vi "displayConfigurableElements.vi"(11 "ConfigurationThisComponent in":refnum<class "ConfigurationTestParameters.lvclass">) -> (3 "ConfigurationThisComponent out":refnum<class "ConfigurationTestParameters.lvclass">)   [LabVIEW 2015, in "ConfigurationTestParameters.lvclass"]
uses:
  ConfigurationTestParameters.lvclass
  <userlib>/Common/Log/Config/Log.ctl
  Typedefs/Supply Voltage Tests.ctl
  Typedefs/Supply Voltage Test.ctl
  Typedefs/ILC Analog Output Tests.ctl
  Typedefs/ILC Static Analog Output Test.ctl
  Typedefs/ILC Analog Output Test.ctl
  Typedefs/Test Values.ctl
  Typedefs/ILC EXC Analog Output Test.ctl
  Typedefs/ILC DAC Analog Output Test.ctl
  Typedefs/ILC Analog Input Tests.ctl
  Typedefs/AI Voltage to NI Voltage.ctl
  Typedefs/ILC Ch0 Analog Input Test.ctl
  Typedefs/Multichannel Analog Input Test.ctl
  Typedefs/Device Configuration Tests.ctl
  Typedefs/1-Wire Test.ctl
  Typedefs/ILC Digital Input Tests.ctl
  Typedefs/ILC Digital Input Test.ctl
  Typedefs/ILC GPI Digital Input Test.ctl
  Typedefs/ILC Digital Output Tests.ctl
  Typedefs/ILC Digital Output Test.ctl
  Typedefs/Digital Signal Level.ctl
  Typedefs/UART Serial Test.ctl
  Typedefs/MUX Settings.ctl
  Typedefs/SSI Serial Test.ctl
  Typedefs/Ground Test.ctl
  Typedefs/ILC Static Digital Output Test.ctl
  Typedefs/Motor Drive Test.ctl
  <userlib>/Common/Log/Log.lvlib
  Typedefs/ILCBTTypedefs.lvlib
panel:
  in  "ctrlRefArrayUsrEvnt":refnum<user-event>
  in  "ConfigTab":T1(tab)
  in  "TestDataLog":T2={"Log Directory"=path "", "Log Filename Base"="", "Max records per file"=1000, "Comment"=""} {"Max records per file" min=100 max=1000000}
  in  "Supply Voltage Tests":T3={"3.3 V Supply"={"Analog Supply DAQ Channel to Read"="AI3", "Digital Supply DAQ Channel to Read"="AI3", "Expected Value"=0.0, "Tolerance"=0.0}, "5 V Supply"={"Analog Supply DAQ Channel to Read"="AI3", "Digital Supply DAQ Channel to Read"="AI3", "Expected Value"=0.0, "Tolerance"=0.0}} {"5 V Supply"."Tolerance" format="%.3f"; "5 V Supply"."Expected Value" format="%.3f"; "3.3 V Supply"."Tolerance" format="%.3f"; "3.3 V Supply"."Expected Value" format="%.3f"}
  in  "Device Configuration Tests":T5
  in  "ILC Digital Input Tests":T7 {"General Purpose Digital Input"."Tachometer Values to Expect"."Stop Value" format="%.6f"; "General Purpose Digital Input"."Tachometer Values to Expect"."Start Value" format="%.6f"; "General Purpose Digital Input"."Frequency Values to Test"."Stop Value" format="%.6f"; "General Purpose Digital Input"."Frequency Values to Test"."Start Value" format="%.6f"}
  in  "ILC Digital Output Tests":T11
  in  "ILC Analog Output Tests":T20 {"DAC"."Tolerance" format="%.4f"; "DAC"."Test Values"."Stop Value" format="%.6f"; "DAC"."Test Values"."Start Value" format="%.6f"; "EXC"."Tolerance" format="%.4f"; "EXC"."Expected Value" format="%.4f"; "BIAS"."Tolerance" format="%.4f"; "BIAS"."Expected Value" format="%.4f"; "ROT"."Tolerance" format="%.4f"; "ROT"."Test Values"."Stop Value" format="%.6f"; "ROT"."Test Values"."Start Value" format="%.6f"; "Vref"."Tolerance" format="%.4f"; "Vref"."Expected Value" format="%.4f"}
  in  "ILC Analog Input Tests":T25 {"5 Channels"."Tolerance" format="%.9f"; "5 Channels"."Test Values"."Stop Value" format="%.6f"; "5 Channels"."Test Values"."Start Value" format="%.6f"; "5 Channels"."PGA Gain Coefficients" max=7; "3 Channels"."Tolerance" format="%.9f"; "3 Channels"."Test Values"."Stop Value" format="%.6f"; "3 Channels"."Test Values"."Start Value" format="%.6f"; "3 Channels"."PGA Gain Coefficients" max=7; "AO Voltage Data"."Bias" min=0.0 max=10.0 format="%.3f"; "AO Voltage Data"."NI Scaling" min=0.0 max=10.0 format="%.3f"; "AO Voltage Data"."Vref" min=0.0 max=10.0 format="%.3f"}
  # "3.3 V Supply"
  # "5 V Supply"
  # "Unique ID Test"
  # "TEDS Status Test"
  # "ms"
  # "Vref"
  # "ROT"
  # "DAC"
  # "BIAS"
  # "EXC"
  # "ms"
  # "AO Voltage Data"
  # "1 Channel"
  # "3 Channels"
  # "5 Channels"
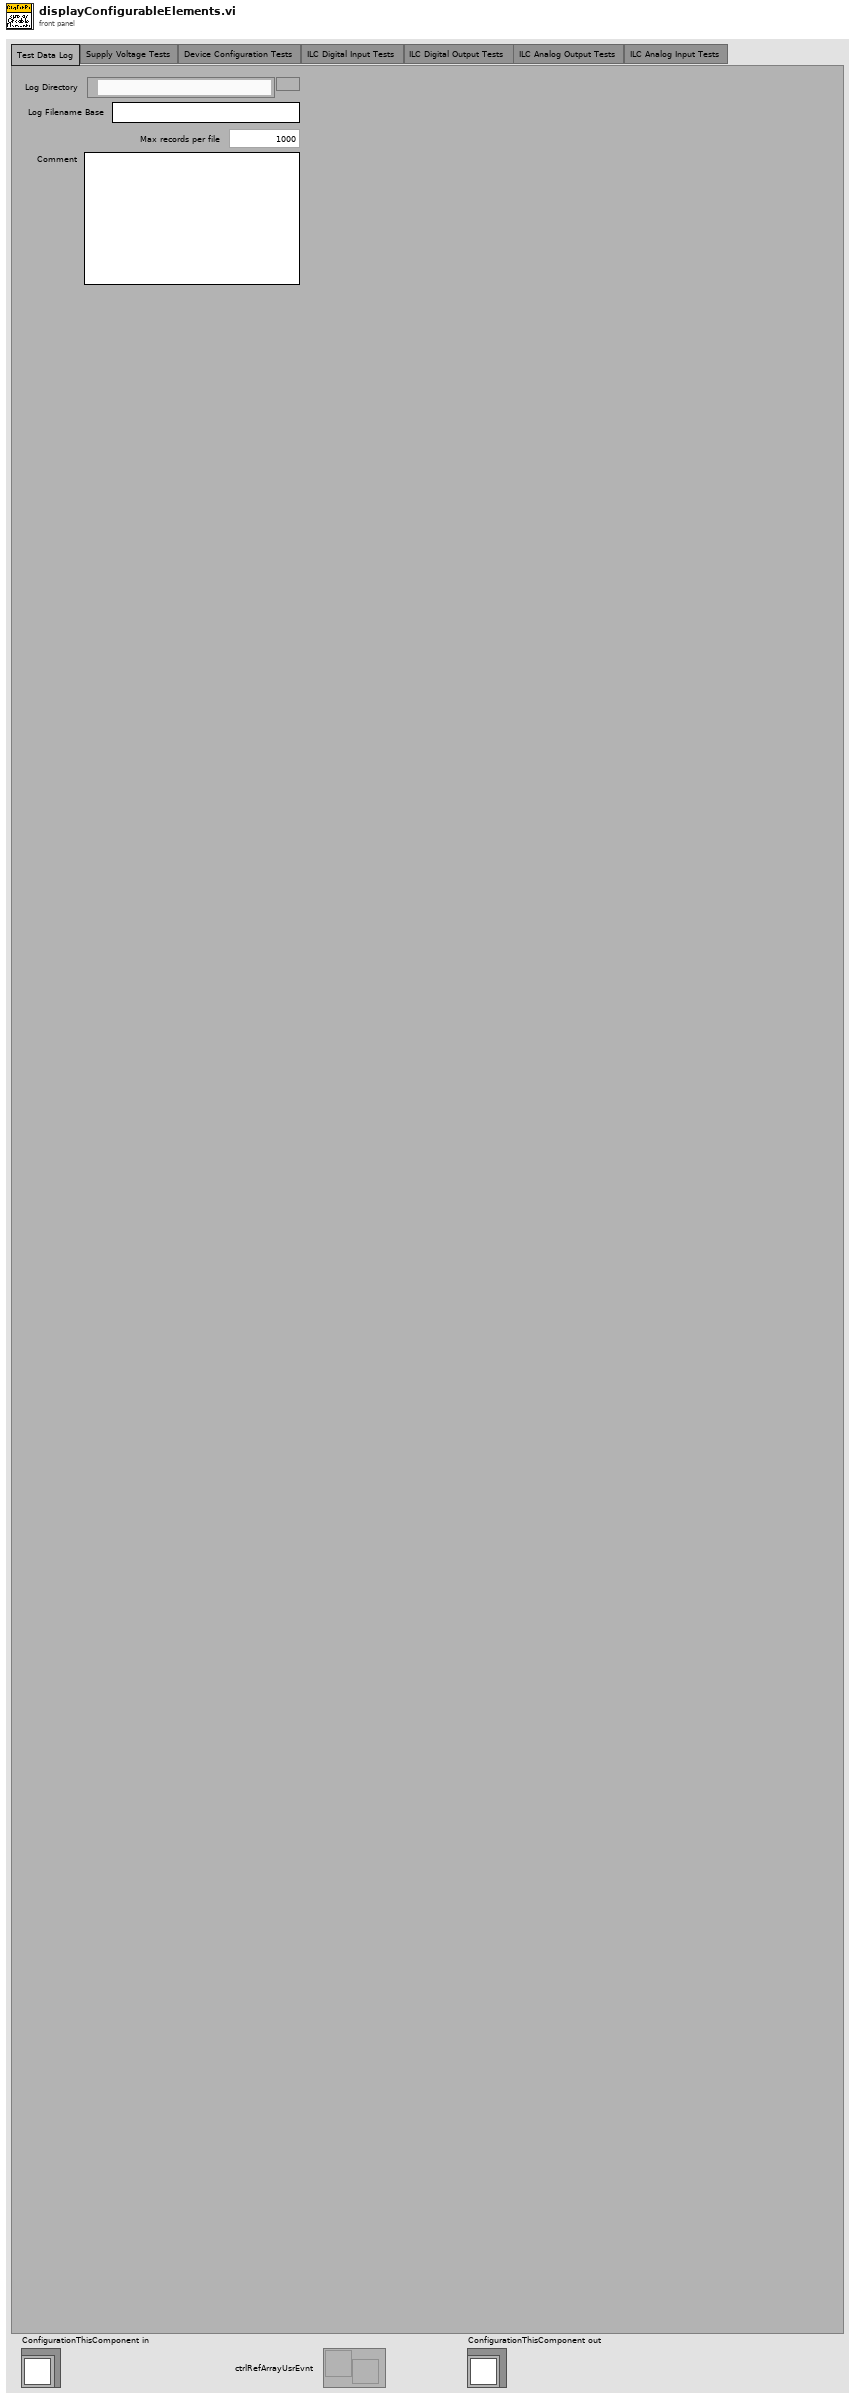
[diagram p1: front panel]
types:
  T1 = enum32{"Test Data Log", "Supply Voltage Tests", "Device Configuration Tests", "ILC Digital Input Tests", "ILC Digital Output Tests", "ILC Analog Output Tests", "ILC Analog Input Tests"}
  T2 = typedef "Log.lvlib/Log.ctl" = cluster{"Log Directory":path, "Log Filename Base":string, "Max records per file":u32, "Comment":string}
  T3 = typedef "ILCBTTypedefs.lvlib/Supply Voltage Tests.ctl" = cluster{"3.3 V Supply":T4, "5 V Supply":T4}
  T4 = typedef "ILCBTTypedefs.lvlib/Supply Voltage Test.ctl" = cluster{"Analog Supply DAQ Channel to Read":refnum<k21>, "Digital Supply DAQ Channel to Read":refnum<k21>, "Expected Value":dbl[unit], "Tolerance":dbl[unit]}
  T5 = typedef "ILCBTTypedefs.lvlib/Device Configuration Tests.ctl" = cluster{"Unique ID Test":T6, "TEDS Status Test":T6}
  T6 = typedef "ILCBTTypedefs.lvlib/1-Wire Test.ctl" = cluster{"Expected Value":string}
  T7 = typedef "ILCBTTypedefs.lvlib/ILC Digital Input Tests.ctl" = cluster{"Limit Switch 1:":T8, "Limit Switch 2:":T8, "General Purpose Digital Input":T9}
  T8 = typedef "ILCBTTypedefs.lvlib/ILC Digital Input Test.ctl" = cluster{"DAQmx Global Channel":refnum<k21>, "High Level Value to Test":enum16{"Low", "High"}, "High Level Value to Expect":enum16{"Low", "High"}, "Low Level Value to Test":enum16{"Low", "High"}, "Low Level Value to Expect":enum16{"Low", "High"}}
  T9 = typedef "ILCBTTypedefs.lvlib/ILC GPI Digital Input Test.ctl" = cluster{"DAQ Channel to Write":refnum<k21>, "Frequency Values to Test":T10, "Tachometer Values to Expect":T10}
  T10 = typedef "ILCBTTypedefs.lvlib/Test Values.ctl" = cluster{"Start Value":dbl, "Stop Value":dbl, "Number of Steps":u16}
  T11 = typedef "ILCBTTypedefs.lvlib/ILC Digital Output Tests.ctl" = cluster{"SSR":T12, "UART Serial Test":T14, "SSI Serial Test":T16, "Ground Test":T17, "Motor Drive Test":T19}
  T12 = typedef "ILCBTTypedefs.lvlib/ILC Digital Output Test.ctl" = cluster{"DAQ Channel to Read":refnum<k21>, "High Level Value to Test":T13, "High Level Value to Expect":T13, "Low Level Value to Test":T13, "Low Level Value to Expect":T13}
  T13 = typedef "ILCBTTypedefs.lvlib/Digital Signal Level.ctl" = enum16{"Low", "High"}
  T14 = typedef "ILCBTTypedefs.lvlib/UART Serial Test.ctl" = cluster{"MUX Settings":T15, "CTS":T12, "TXD":T12, "RTS":T12, "RXD":T12}
  T15 = typedef "ILCBTTypedefs.lvlib/MUX Settings.ctl" = cluster{"MUX_AO":T13, "MUX_A1":T13}
  T16 = typedef "ILCBTTypedefs.lvlib/SSI Serial Test.ctl" = cluster{"MUX Settings":T15, "Out_SS":T12, "Out_SDI":T12, "Out_SCLK":T12, "Reset":T12}
  T17 = typedef "ILCBTTypedefs.lvlib/Ground Test.ctl" = cluster{"MUX Settings":T15, "Gnd1":T18, "Gnd2":T18, "Gnd3":T18, "Gnd4":T18}
  T18 = typedef "ILCBTTypedefs.lvlib/ILC Static Digital Output Test.ctl" = cluster{"DAQ Channel to Read":refnum<k21>, "Expected Signal Level":T13}
  T19 = typedef "ILCBTTypedefs.lvlib/Motor Drive Test.ctl" = cluster{"MUX Settings":T15, "SM_CW":T12, "SM_CCW":T12, "SM_GPI":T12}
  T20 = typedef "ILCBTTypedefs.lvlib/ILC Analog Output Tests.ctl" = cluster{"Delay Between Test Steps":u16, "Vref":T21, "ROT":T22, "BIAS":T21, "EXC":T23, "DAC":T24}
  T21 = typedef "ILCBTTypedefs.lvlib/ILC Static Analog Output Test.ctl" = cluster{"DAQ Channel to Read":refnum<k21>, "Expected Value":dbl[unit], "Tolerance":dbl[unit]}
  T22 = typedef "ILCBTTypedefs.lvlib/ILC Analog Output Test.ctl" = cluster{"DAQ Channel to Read":refnum<k21>, "Test Values":T10, "Tolerance":dbl[unit]}
  T23 = typedef "ILCBTTypedefs.lvlib/ILC EXC Analog Output Test.ctl" = cluster{"EXC1 DAQ Channel to Read":refnum<k21>, "EXC2 DAQ Channel to Read":refnum<k21>, "EXC3 DAQ Channel to Read":refnum<k21>, "EXC4 DAQ Channel to Read":refnum<k21>, "Expected Value":dbl[unit], "Tolerance":dbl[unit]}
  T24 = typedef "ILCBTTypedefs.lvlib/ILC DAC Analog Output Test.ctl" = cluster{"DAC1 DAQ Channel to Read":refnum<k21>, "DAC2 DAQ Channel to Read":refnum<k21>, "DAC3 DAQ Channel to Read":refnum<k21>, "DAC4 DAQ Channel to Read":refnum<k21>, "Test Values":T10, "Tolerance":dbl[unit]}
  T25 = typedef "ILCBTTypedefs.lvlib/ILC Analog Input Tests.ctl" = cluster{"CH13 DAQ Channel to Write":refnum<k21>, "CH24 DAQ Channel to Write":refnum<k21>, "AO Voltage Data":T26, "Delay Between Test Steps":u16, "1 Channel":T27, "3 Channels":T28, "5 Channels":T28}
  T26 = typedef "ILCBTTypedefs.lvlib/AI Voltage to NI Voltage.ctl" = cluster{"ADC Bit Count":u16, "Vref":dbl[unit], "NI Scaling":dbl, "Bias":dbl[unit]}
  T27 = typedef "ILCBTTypedefs.lvlib/ILC Ch0 Analog Input Test.ctl" = cluster{"ADC Configurations":string[], "Value to Expect":i32, "Tolerance":i32}
  T28 = typedef "ILCBTTypedefs.lvlib/Multichannel Analog Input Test.ctl" = cluster{"ADC Configurations":string[], "PGA Gain Coefficients":u16[], "Test Values":T10, "Tolerance":dbl[unit]}
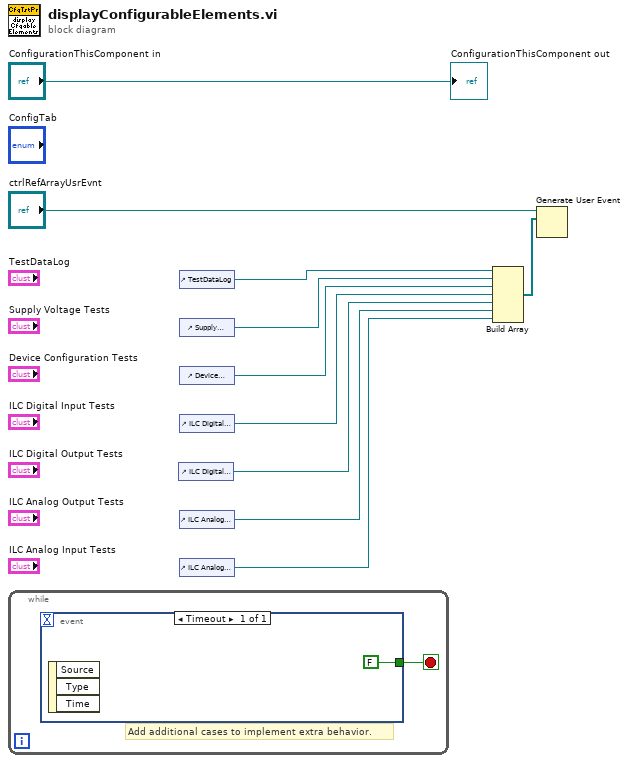
[diagram p0: block diagram]
diagram:
  n1 = while {
    stop <- w11 stop-if-true
    # "Add additional cases to implement extra behavior."
    n2 = event shown="[0] Timeout" {
      selector: _ -> [_]
      dyn-events: _ -> [_]
      timeout: _ -> [_]
      tunnel: [FALSE] -> w11
      event Timeout {
        n3 = event-data() -> ()  [unwired: 1 in, 3 out]
      }
    }
  }
  n4 = control-ref of="ILC Digital Output Tests"() -> (w3:refnum<vi>)
  n5 = control-ref of="TestDataLog"() -> (w7:refnum<vi>)
  n6 = control-ref of="Supply Voltage Tests"() -> (w6:refnum<vi>)
  n7 = control-ref of="Device Configuration Tests"() -> (w5:refnum<vi>)
  n8 = control-ref of="ILC Digital Input Tests"() -> (w4:refnum<vi>)
  n9 = control-ref of="ILC Analog Output Tests"() -> (w2:refnum<vi>)
  n10 = control-ref of="ILC Analog Input Tests"() -> (w1:refnum<vi>)
  n11 = Build Array(w7, w6, w5, w4, w3, w2, w1) -> (w8:refnum<vi>[])
  n12 = Generate User Event(user event="ctrlRefArrayUsrEvnt", event data cluster=w8) -> ()  [unwired: 2 in, 2 out]
  "ConfigurationThisComponent out" <- "ConfigurationThisComponent in"
